vi "DT_Triangle Manager_Format Edge_Double Side.vi"(4 "right bottom tri":i32, 5 "left bottom tri":i32, 6 "right top tri":i32, 7 "left top tri":i32, 9 "start triangle":i32, 10 "right point":i32, 11 "left point":i32) -> (2 "Second Triangle":i32[](array[numeric]), 3 "First Triangle":i32[](array[numeric]))   [LabVIEW 2020, in "NI_AAL_Geometry.lvlib"]
uses:
  <vilib>/Analysis/NI_AAL_Geometry.lvlib
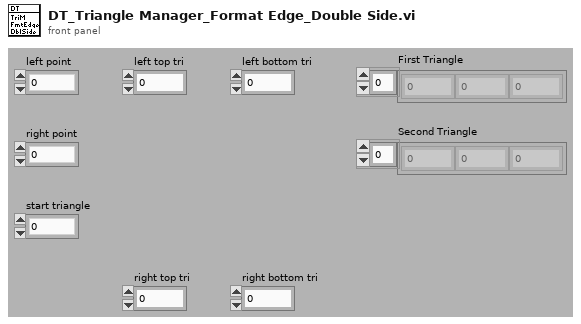
[diagram p1: front panel]
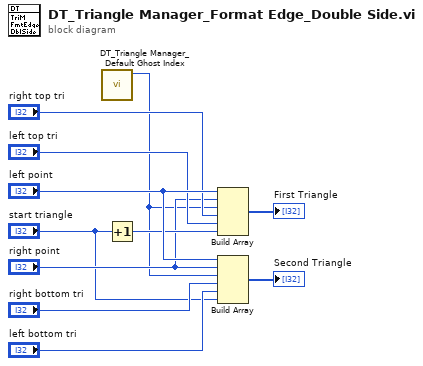
[diagram p0: block diagram]
diagram:
  n1 = call <vilib>:"DT_Triangle Manager_Default Ghost Index.vi"() -> ("ghost index"=w1:i32)  [unwired: 11 out]
  n2 = Increment(x="start triangle") -> (x+1=w8:i32)
  n3 = Build Array("left point", "right point", w1, "right top tri", "left top tri", w8) -> (→"First Triangle":i32[])
  n4 = Build Array("left point", "right point", w1, "right bottom tri", "left bottom tri", "start triangle") -> (→"Second Triangle":i32[])
